vi "Flow Module (Main).vi"(7 "Name of Parent Panel":string="Main.vi", 9 "New Center Coords":T1={"Horizontal"=470, "Vertical"=200}, 10 "Config":variant, 11 "Main UI Message Queue":refnum<queue>) -> ()   [LabVIEW 2018, in "Flow Module.lvlib"]
doc: "This Continuous Measurement sample project is based on the Queued Message Handler template.\n\nThe Event Handling Loop generates messages based on user interface actions.\n\nThe Message Handling Loop processes messages generated by the Event Handling Loop, or by other messages. There are also Acquisition and Logging message handling loop subVIs, and a chart updating loop."
uses:
  Flow Module.lvlib
  support/Message Queue/Message Cluster.ctl
  <vilib>/Utility/miscctls.llb/LVPoint32TypeDef.ctl
  controls/UI State.ctl
  Feed Module/Controls/Flow Module Config Cluster.ctl
  Feed Module/Controls/Flow Module Settings Cluster.ctl
  Mettler Toledo/Controls/Settings Cluster.ctl
  Feed Module/Controls/Flow Module State Cluster.ctl
  Feed Module/Controls/Flow Module Display.ctl
  support/Message Queue/Enqueue Message (Single).vi
  support/User Event - Stop/User Event - Stop.lvlib
  support/Message Queue/Message Queue.lvlib
  support/Support Library.lvlib
  Measure Instrument/Flow Module Engine.lvlib
  Mettler Toledo/Mettler Toledo.lvlib
  support/Command Log VIs/Command Logging.lvlib
panel:
  in  "Settings Button":bool
  out "C":dbl format="%5.2f"
  out "kg/m^3":dbl format="%6.1f"
  out "ScanCode":i16
  out "g/min":dbl format="%4.2f"
  out "Log File path":path
  out "Status":string
  in  "Exit":bool
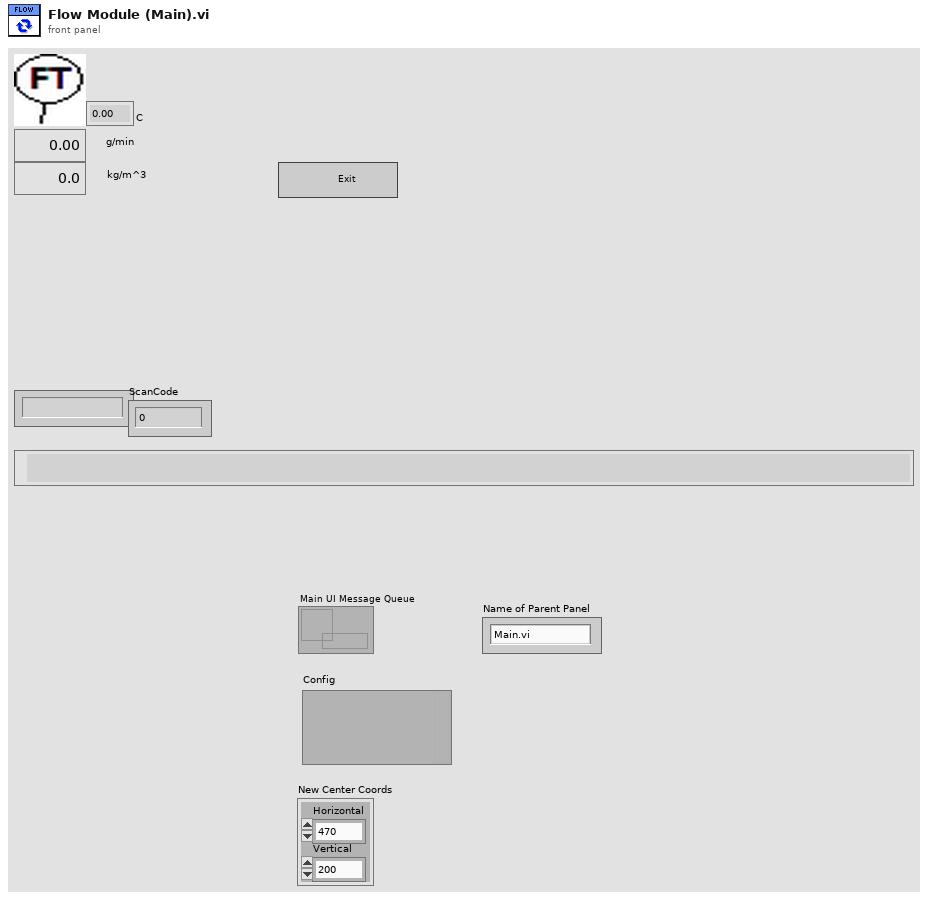
[diagram p1: front panel]
types:
  T1 = typedef "LVPoint32TypeDef.ctl" = cluster{"Horizontal":i32, "Vertical":i32}
  T2 = typedef "Flow Module.lvlib/Flow Module State Cluster.ctl" = cluster{"Flow Module Config":T3}
  T3 = typedef "Flow Module.lvlib/Flow Module Config Cluster.ctl" = cluster{"GUID":string, "Drop Coords":T1, "Process Name":string, "Queue Name":string, "Settings":T4, "Load Count":i32}
  T4 = typedef "Flow Module.lvlib/Flow Module Settings Cluster.ctl" = cluster{"Cycle Period":dbl, "Bronkhorst M13":T5, "Flow Meter Type":string, "Bronkhorst M14":T5}
  T5 = typedef "Mettler Toledo.lvlib/Settings Cluster.ctl" = cluster{"VISA resource name":refnum<visa-resource-name>, "Simulated?":bool}
  T6 = typedef "UI State.ctl" = enum16{"Idle", "Acquiring and Logging", "Waiting for Exit", "Waiting for Exit (Acq Stopped)", "Waiting for Exit (Log Stopped)", "Waiting for Stop", "Waiting for Stop (Acq Stopped)", "Waiting for Stop (Log Stopped)"}
  T7 = typedef "Flow Module.lvlib/Flow Message Queues.ctl" = cluster{"Flow UI":refnum<queue>, "Flow Engine":refnum<queue>, "Flow Display":refnum<queue>}
  T8 = typedef "Flow Module.lvlib/Flow Module Display.ctl" = cluster{"Flow Value":dbl, "Cycle Period":dbl, "Density":dbl, "Temp":dbl}
  T9 = cluster{"Shift":bool, "Ctrl":bool, "Alt":bool, "Cmd":bool, "Opt":bool}
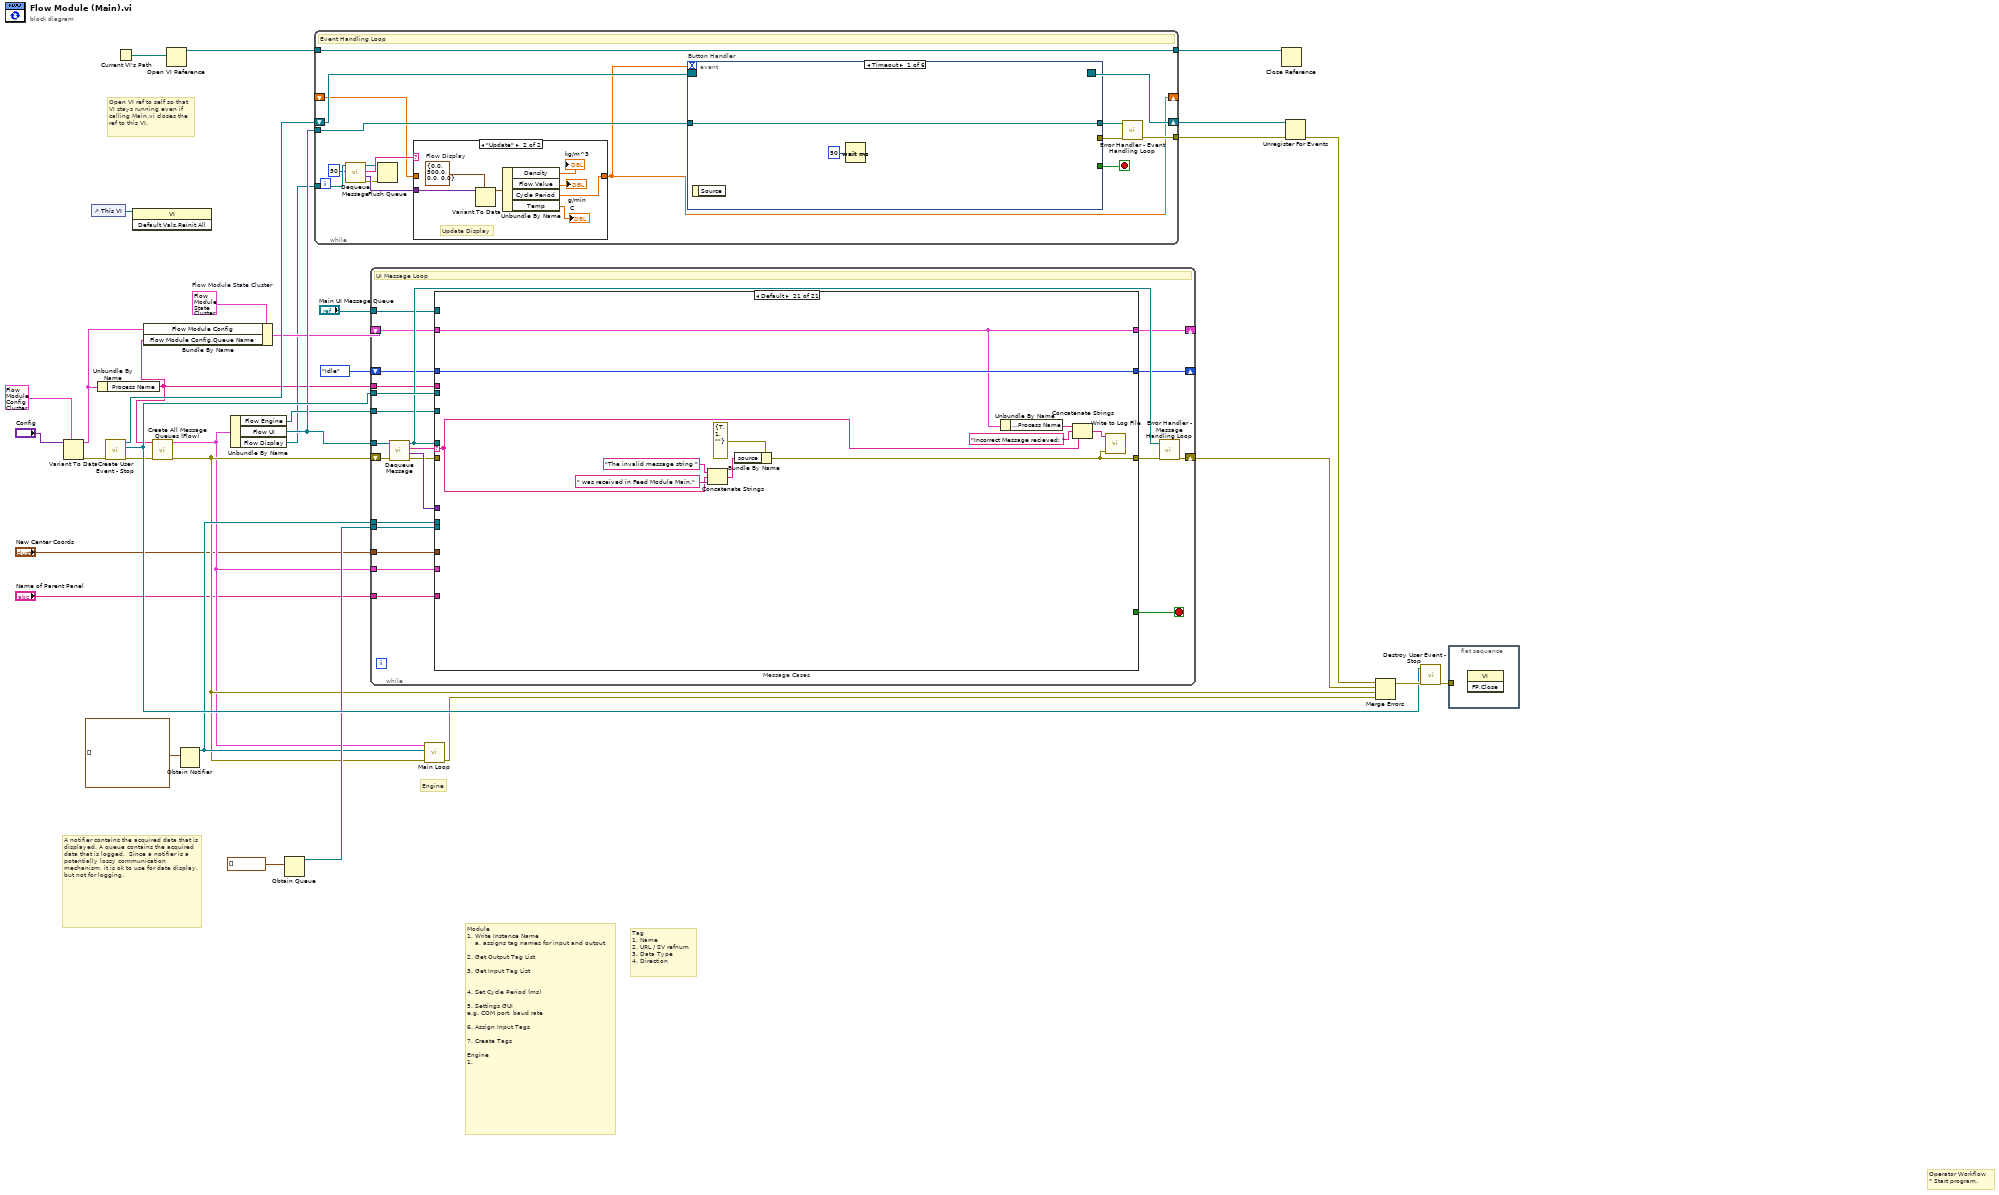
[diagram p0: block diagram]
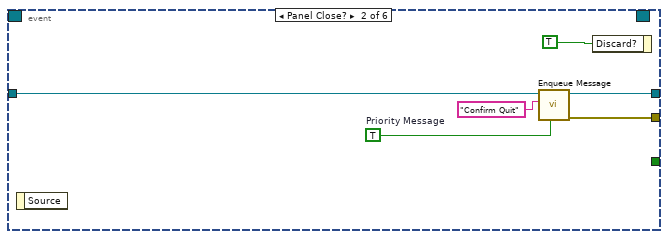
[diagram p3: hidden frame]
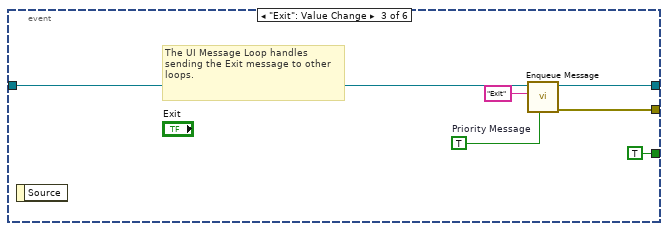
[diagram p4: hidden frame]
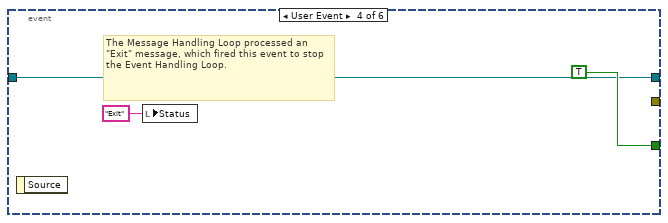
[diagram p5: hidden frame]
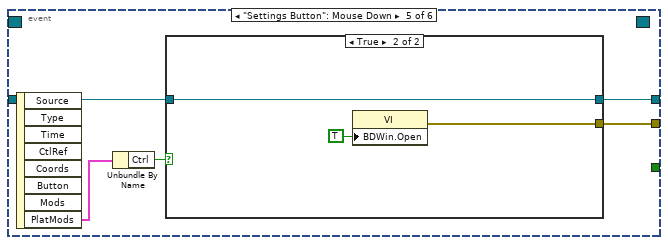
[diagram p6: hidden frame]
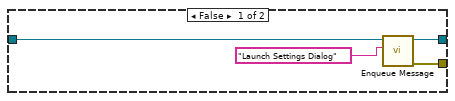
[diagram p7: hidden frame]
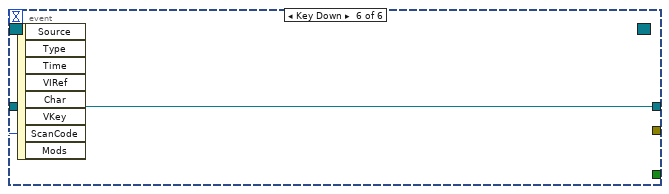
[diagram p8: hidden frame]
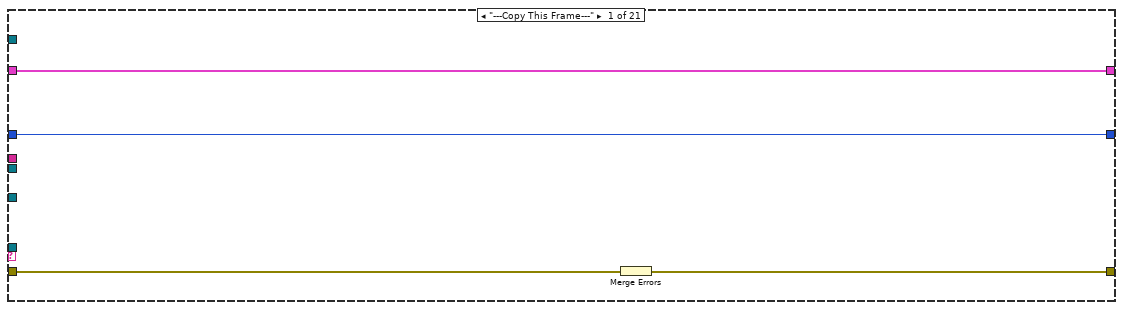
[diagram p9: hidden frame]
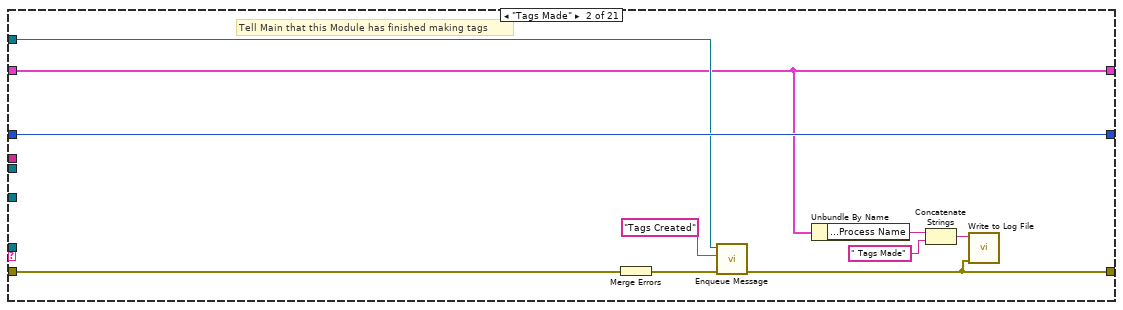
[diagram p10: hidden frame]
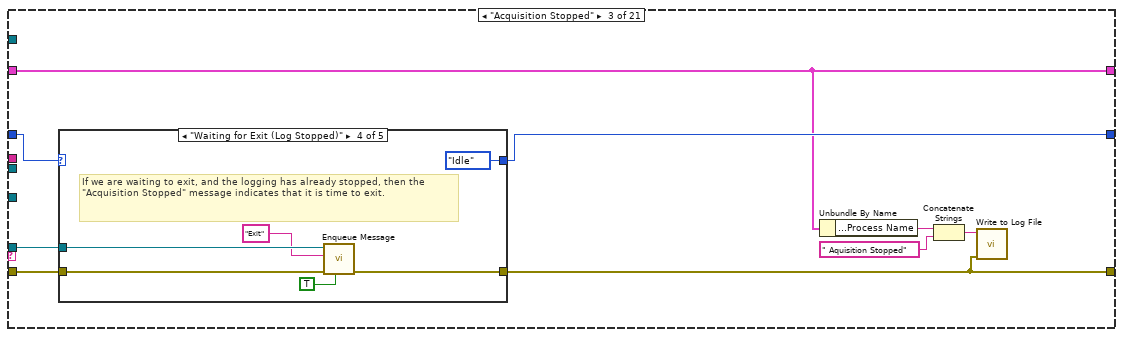
[diagram p11: hidden frame]
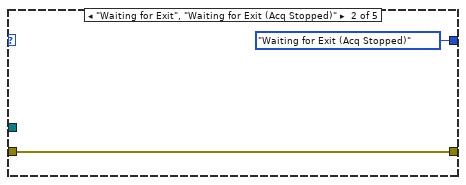
[diagram p13: hidden frame]
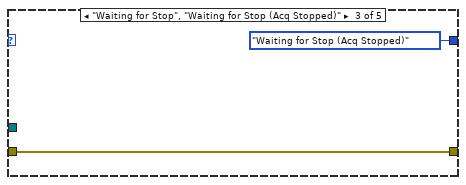
[diagram p14: hidden frame]
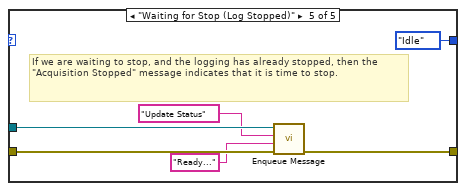
[diagram p15: hidden frame]
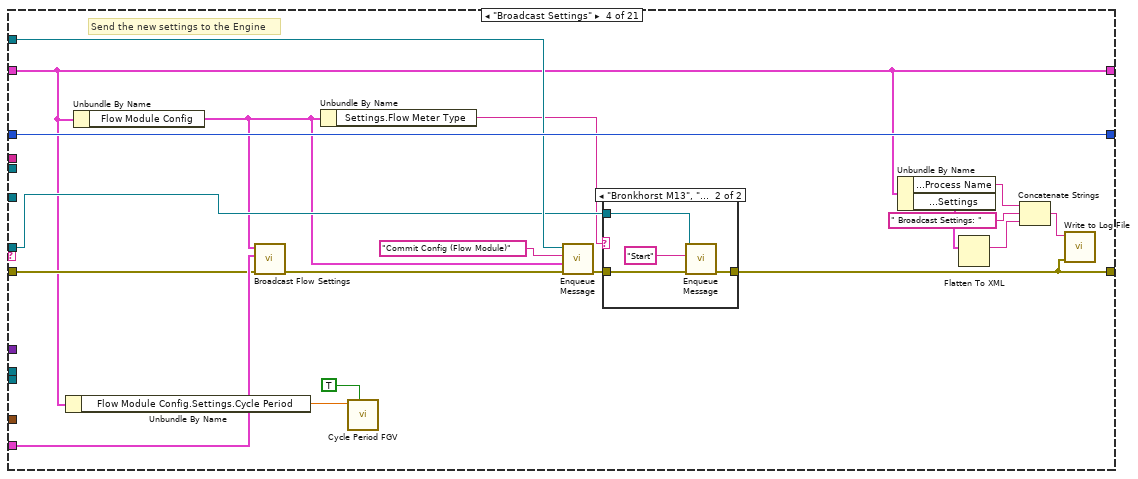
[diagram p16: hidden frame]
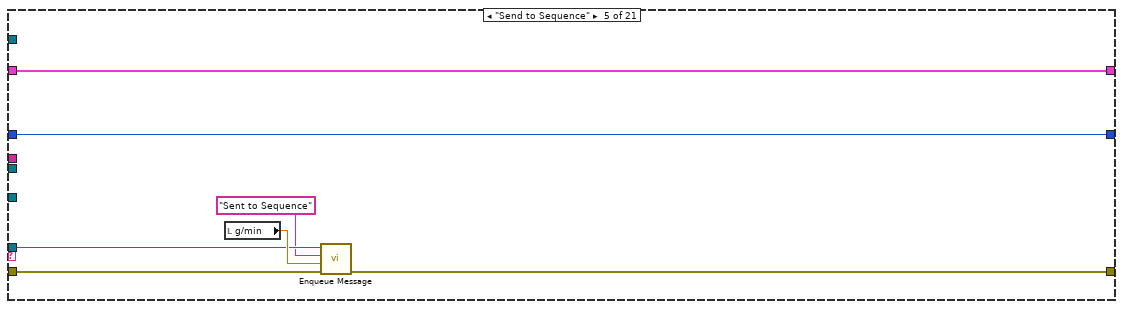
[diagram p18: hidden frame]
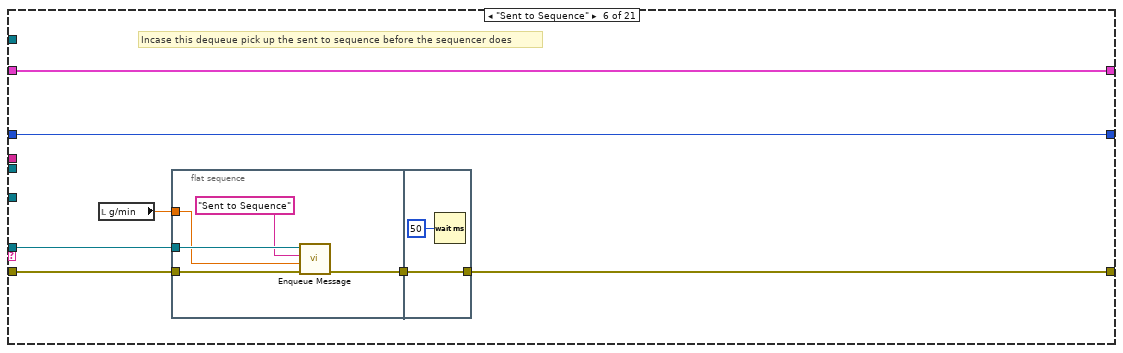
[diagram p19: hidden frame]
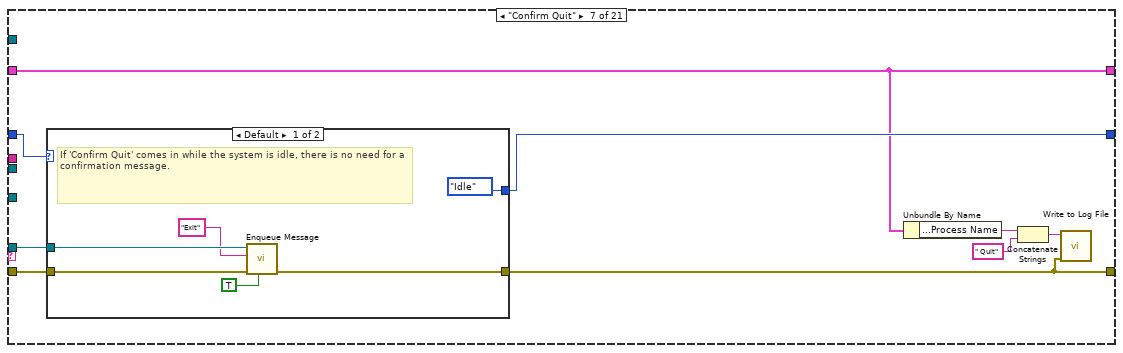
[diagram p20: hidden frame]
diagram:
  w2 = T2 {"Flow Module Config"={"GUID"="PID1-Mettler Toledo Scale 1", "Drop Coords"={"Horizontal"=0, "Vertical"=0}, "Process Name"="PID1-Setpoint", "Queue Name"="", "Settings"={"Cycle Period"=500.0, "Bronkhorst M13"={"VISA resource name"="", "Simulated?"=FALSE}, "Flow Meter Type"="", "Bronkhorst M14"={"VISA resource name"="", "Simulated?"=FALSE}}, "Load Count"=0}}  # Flow Module State Cluster
  # "Open VI ref to self so that\nVI stays running even if\ncalling Main.vi closes the\nref to this VI."
  # "Engine"
  # "Operator Workflow\n* Start program."
  # "Module \n1. Write Instance Name\n    a. assigns tag names for input and output\n\n2. Get Output Tag List\n\n3. Get Input Tag List\n\n\n4. Set Cycle Period (ms)\n\n5. Settings GUI\ne.g. COM port, baud rate\n\n6. Assign Input Tags\n\n7. Create Tags\n\nEngine\n1."
  # "Tag\n1. Name\n2. URL / SV refnum\n3. Data Type\n4. Direction"
  # "A notifier contains the acquired data that is displayed. A queue contains the acquired data that is logged.  Since a notifier is a potentially lossy communication mechanism, it is ok to use for data display, but not for logging."
  n1 = Variant To Data(type=T3 {"GUID"="", "Drop Coords"={"Horizontal"=0, "Vertical"=0}, "Process Name"="", "Queue Name"="", "Settings"={"Cycle Period"=500.0, "Bronkhorst M13"={"VISA resource name"="", "Simulated?"=FALSE}, "Flow Meter Type"="", "Bronkhorst M14"={"VISA resource name"="", "Simulated?"=FALSE}}, "Load Count"=0} ("Feed Module Config"), Variant="Config") -> (data=w11:T3, error out=w15:errorcluster)  [unwired: 1 in]
  n2 = control-ref of="This VI"() -> (w10:refnum<vi>)
  n3 = Unbundle By Name(w11) -> ("Process Name"=w1:string)
  n4 = call "Create User Event - Stop.vi"("error in (no error)"=w15) -> ("error out"=w8:errorcluster, "User Event - Stop"=w30:refnum<user-event>, "Stop Event Registration Refnum"=w31:refnum<event-registration>)  [unwired: 8 in]
  n5 = Current VI's Path() -> (path=w17:path)
  n6 = invoke class="VI" method="Default Vals.Reinit All"(reference=w10) -> ()  [unwired: 2 in, 3 out]
  n7 = Bundle By Name(cluster=w2, "Flow Module Config"=w11, "Flow Module Config.Queue Name"=w1) -> (w16:T2)
  n8 = call "Create All Message Queues (Flow).vi"("error in (no error)"=w8, "Process Name"=w1) -> ("error out"=w7:errorcluster, "Message Queues"=w6:T7)  [unwired: 8 in]
  n9 = Open VI Reference(vi path=w17) -> (vi reference=w18:refnum<vi>)  [unwired: 5 in, 1 out]
  n10 = Obtain Notifier(notification data type=waveform(dbl)[] []) -> (notifier out=w20:refnum<notifier>)  [unwired: 3 in, 2 out]
  n11 = Unbundle By Name(w6) -> ("Flow Engine"=w23:refnum<queue>, "Flow UI"=w27:refnum<queue>, "Flow Display"=w12:refnum<queue>)
  n12 = Obtain Queue(element data type=waveform(dbl)[] []) -> (queue out=w22:refnum<queue>)  [unwired: 4 in, 2 out]
  n13 = while {
    tunnel: w27 -> [w44]
    tunnel: [w46] -> w33
    shift-right: [w45] -> w28
    shift-left: w31 -> [w50]
    tunnel: [w43] -> w19
    tunnel: w18 -> [w43]
    tunnel: w12 -> [w42]
    shift-right: [w39] -> _
    shift-left: _ -> [w38]
    stop <- w49 stop-if-true
    # "Event Handling Loop"
    n14 = call "Dequeue Message.vi"("timeout in ms (-1)"=50, "Message Queue"=w42) -> ("error out"=w35:errorcluster, "Message Data"=w40:variant, "Message"=w41:string, "dup Message Queue"=w36:refnum<queue>)  [unwired: 6 in]
    n15 = Flush Queue(queue=w36, error in (no error)=w35) -> ()  [unwired: 3 out]
    n16 = case shown="\"Update\"" w41 {
      tunnel: w40 -> [_ w58]
      tunnel: [w51 w55] -> w39
      tunnel: w38 -> [w51 _]
      frame "False", Default {
      }
      frame "Update" {
        w54 = T8 {"Flow Value"=0.0, "Cycle Period"=500.0, "Density"=0.0, "Temp"=0.0}  # Flow Display
        # "Update Display"
        n17 = Variant To Data(type=w54, Variant=w58) -> (data=w57:T8)  [unwired: 1 in, 1 out]
        n18 = Unbundle By Name(w57) -> ("Density"=→"kg/m^3":dbl, "Flow Value"=→"g/min":dbl, "Cycle Period"=w55:dbl, "Temp"=→"C":dbl)
      }
    }
    n19 = event "Button Handler" shown="[0] Timeout" {
      selector: w50 -> [_ _ _ _ _ _]
      dyn-events: [_ _ _ _ _ _] -> w45
      timeout: w39 -> [_ _ _ _ _ _]
      tunnel: [_ _ TRUE ("Discard?") TRUE ("Discard?") _ _] -> w49
      tunnel: w44 -> [w60 w63 w67 w73 w78 w88]
      tunnel: [_ w61 w72 _ w80 _] -> w47
      tunnel: [w60 w62 w70 w73 w79 w88] -> w48
      event Timeout {
        n20 = event-data() -> ()  [unwired: 1 in, 1 out]
        n21 = Wait (ms)(milliseconds to wait=u32 50) -> ()  [unwired: 1 out]
      }
      event Panel Close? {
        w64 = TRUE  # Priority Message
        n22 = event-data() -> ()  [unwired: 1 in, 1 out]
        n23 = call-poly "Enqueue Message.vi"("Priority Message? (F)"=w64, "Message"="Confirm Quit", "Message Queue"=w63) -> ("error out"=w61:errorcluster, "dup Message Queue"=w62:refnum<queue>)  [unwired: 7 in]
        n24 = event-data("Discard?"=TRUE) -> ()  [unwired: 1 in, 1 out]
      }
      event "Exit": Value Change {
        w68 = TRUE  # Priority Message
        # "The UI Message Loop handles sending the Exit message to other loops."
        n25 = event-data() -> ()  [unwired: 1 in, 1 out]
        n26 = call-poly "Enqueue Message.vi"("Priority Message? (F)"=w68, "Message"="Exit", "Message Queue"=w67) -> ("error out"=w72:errorcluster, "dup Message Queue"=w70:refnum<queue>)  [unwired: 7 in]
      }
      event User Event {
        # "The Message Handling Loop processed an \"Exit\" message, which fired this event to stop the Event Handling Loop."
        n27 = event-data() -> ()  [unwired: 1 in, 1 out]
        n28 = local write "Status"("Exit" ("Exit String")) -> ()
      }
      event "Settings Button": Mouse Down {
        n29 = event-data() -> ("PlatMods"=w77:T9)  [unwired: 1 in, 7 out]
        n30 = Unbundle By Name(w77) -> ("Ctrl"=w76:bool)
        n31 = case shown="True" w76 {
          tunnel: [w84 w85] -> w80
          tunnel: [w83 w86] -> w79
          tunnel: w78 -> [w82 w86]
          frame False {
            n32 = call-poly "Enqueue Message.vi"("Message"="Launch Settings Dialog", "Message Queue"=w82) -> ("error out"=w84:errorcluster, "dup Message Queue"=w83:refnum<queue>)  [unwired: 8 in]
          }
          frame True {
            n33 = property class="VI"("BDWin.Open"=TRUE ("Block Diagram Window:Open")) -> (error out=w85:errorcluster)  [unwired: 2 in, 1 out]
          }
        }
      }
      event Key Down {
        n34 = event-data() -> ("ScanCode"=→"ScanCode":i16)  [unwired: 1 in, 7 out]
      }
    }
    n35 = call "Error Handler - Event Handling Loop.vi"("error in (no error)"=w47, "Message Queue"=w48) -> ("dup error in"=w46:errorcluster)  [unwired: 8 in, 1 out]
  }
  n36 = while {
    tunnel: w27 -> [w106]
    tunnel: w30 -> [w110]
    shift-right: [w102] -> w34
    shift-left: w7 -> [w109]
    shift-right: [w93] -> _
    shift-left: w16 -> [w95]
    tunnel: w20 -> [w105]
    tunnel: w22 -> [w104]
    shift-right: [w99] -> _
    shift-left: UI_State."Idle" ("UI State") -> [w100]
    tunnel: w23 -> [w98]
    tunnel: w6 -> [w97]
    tunnel: "Main UI Message Queue" -> [w94]
    tunnel: w1 -> [w92]
    tunnel: "New Center Coords" -> [w91]
    tunnel: "Name of Parent Panel" -> [w90]
    stop <- w111 stop-if-true
    # "UI Message Loop"
    n37 = call "Dequeue Message.vi"("error in (no error)"=w109, "Message Queue"=w106) -> ("error out"=w96:errorcluster, "Message Data"=w107:variant, "Message"=w108:string, "dup Message Queue"=w101:refnum<queue>)  [unwired: 6 in]
    n38 = case "Message Cases" shown="Default" w108 {
      selector: w108 -> [_ _ _ _ _ _ _ _ _ _ _ _ _ _ _ _ _ _ _ _ w436]
      tunnel: w101 -> [_ _ w131 w163 w178 w186 w205 _ w246 w260 w282 _ w321 w338 w355 w383 _ _ w425 _ _]
      tunnel: w96 -> [w115 w125 w132 w167 w181 w188 w204 w230 w241 w264 w281 w307 w317 w335 w356 w382 w389 w408 w420 w434 _]
      tunnel: [w114 w117 w127 w156 w180 w187 w199 w231 w236 w251 w266 w307 w309 w328 w351 w378 w394 w401 w412 w435 w437] -> w103
      tunnel: [_ _ _ _ _ _ _ _ _ _ TRUE _ _ _ _ _ _ _ _ _ _] -> w111
      tunnel: w107 -> [_ _ _ _ _ _ _ w233 _ w263 w271 _ _ _ _ _ _ _ _ w433 _]
      tunnel: w110 -> [_ _ _ _ _ _ _ _ _ _ w292 _ _ _ _ _ _ _ _ _ _]
      tunnel: w95 -> [w112 w116 w126 w155 w182 w189 w198 w228 w235 w250 w265 w304 w308 w340 w350 w377 w387 w400 w411 w428 w442]
      tunnel: w105 -> [_ _ _ _ _ _ _ _ _ _ w290 _ _ _ _ _ _ _ _ _ _]
      tunnel: w104 -> [_ _ _ _ _ _ _ _ _ _ w286 _ _ _ _ _ _ _ _ _ _]
      tunnel: w100 -> [w113 w124 w134 w171 w183 w190 w206 w229 w242 w255 w279 _ _ w344 w358 _ _ _ w421 w429 w446]
      tunnel: [w113 w124 w133 w171 w183 w190 w203 w229 w243 w255 w278 UI_State."Idle" ("UI State") UI_State."Idle" ("UI State") w344 w357 UI_State."Acquiring and Logging" ("UI State") UI_State."Acquiring and Logging" ("UI State") UI_State."Acquiring and Logging" ("UI State") w422 w429 w446] -> w99
      tunnel: w98 -> [_ _ _ _ _ _ _ _ _ _ w285 _ _ _ _ _ w392 w406 w419 _ _]
      tunnel: w97 -> [_ _ _ w170 _ _ _ _ _ _ _ _ _ _ _ _ _ _ _ _ _]
      tunnel: w94 -> [_ w121 _ w164 _ _ _ _ _ _ w270 _ _ w341 _ _ _ _ _ _ _]
      tunnel: [w112 w116 w126 w155 w182 w189 w198 w228 w235 w250 w265 w304 w308 w329 w350 w377 w387 w400 w411 w428 w442] -> w93
      tunnel: w92 -> [_ _ _ _ _ _ _ _ _ _ _ _ w315 _ _ _ _ w405 _ _ _]
      tunnel: w91 -> [_ _ _ _ _ _ _ _ _ _ _ _ w314 _ _ _ _ _ _ _ _]
      tunnel: w90 -> [_ _ _ _ _ _ _ _ _ _ _ _ w313 _ _ _ _ _ _ _ _]
      frame "---Copy This Frame---" {
        # "Duplicate this frame when creating new messages.  Change this comment in the duplicated frame to describe this message."
        n39 = Merge Errors(w115) -> (w114:errorcluster)
      }
      frame "Tags Made" {
        # "Tell Main that this Module has finished making tags"
        # "Duplicate this frame when creating new messages.  Change this comment in the duplicated frame to describe this message."
        n40 = Merge Errors(w125) -> (w122:errorcluster)
        n41 = call-poly "Enqueue Message.vi"("error in (no error)"=w122, "Message"="Tags Created", "Message Queue"=w121) -> ("error out"=w117:errorcluster)  [unwired: 7 in, 1 out]
        n42 = Unbundle By Name(w116) -> ("Flow Module Config.Process Name"=w120:string)
        n43 = Concatenate Strings(w120, " Tags Made" ("text")) -> (w118:string)
        n44 = call "Write to Log File.vi"("error in"=w117, "text"=w118) -> ()  [unwired: 9 in, 1 out]
      }
      frame "Acquisition Stopped" {
        # "Logic for determining what action to take when the acquisition has stopped."
        n45 = case shown="\"Waiting for Exit (Log Stopped)\"" w134 {
          selector: w134 -> [w136 _ _ _ _]
          tunnel: [w136 UI_State."Waiting for Exit (Acq Stopped)" ("UI State") UI_State."Waiting for Stop (Acq Stopped)" ("UI State") UI_State."Idle" ("UI State") UI_State."Idle" ("UI State")] -> w133
          tunnel: w132 -> [w135 w137 w139 w145 w151]
          tunnel: [w135 w137 w139 w144 w150] -> w127
          tunnel: w131 -> [_ _ _ w143 w149]
          frame Default {
          }
          frame "Waiting for Exit", "Waiting for Exit (Acq Stopped)" {
          }
          frame "Waiting for Stop", "Waiting for Stop (Acq Stopped)" {
          }
          frame "Waiting for Exit (Log Stopped)" {
            # "If we are waiting to exit, and the logging has already stopped, then the \"Acquisition Stopped\" message indicates that it is time to exit."
            n46 = call-poly "Enqueue Message.vi"("Priority Message? (F)"=TRUE, "error in (no error)"=w145, "Message"="Exit", "Message Queue"=w143) -> ("error out"=w144:errorcluster)  [unwired: 6 in, 1 out]
          }
          frame "Waiting for Stop (Log Stopped)" {
            # "If we are waiting to stop, and the logging has already stopped, then the \"Acquisition Stopped\" message indicates that it is time to stop."
            n47 = call-poly "Enqueue Message.vi"("error in (no error)"=w151, "Message Data"="Ready..." ("Message"), "Message"="Update Status", "Message Queue"=w149) -> ("error out"=w150:errorcluster)  [unwired: 6 in, 1 out]
          }
        }
        n48 = Unbundle By Name(w126) -> ("Flow Module Config.Process Name"=w130:string)
        n49 = Concatenate Strings(w130, " Aquisition Stopped" ("text")) -> (w128:string)
        n50 = call "Write to Log File.vi"("error in"=w127, "text"=w128) -> ()  [unwired: 9 in, 1 out]
      }
      frame "Broadcast Settings" {
        # "Send the new settings to the Engine"
        # "Send the 'Update Settings' message to the Logging and Acquisition message loops."
        n51 = Unbundle By Name(w155) -> ("Flow Module Config.Settings.Cycle Period"=w168:dbl)
        n52 = Unbundle By Name(w155) -> ("Flow Module Config"=w160:T3)
        n53 = call "Broadcast Flow Settings.vi"("error in (no error)"=w167, "Message Queues"=w170, "Flow Module Config"=w160) -> ("error out"=w165:errorcluster)  [unwired: 8 in]
        n54 = Unbundle By Name(w160) -> ("Settings.Flow Meter Type"=w161:string)
        n55 = call "Cycle Period FGV.vi"("Write"=TRUE, "Cycle Period In (ms)"=w168) -> ()  [unwired: 8 in, 2 out]
        n56 = call-poly "Enqueue Message.vi"("error in (no error)"=w165, "Message Data"=w160, "Message"="Commit Config (Flow Module)", "Message Queue"=w164) -> ("error out"=w162:errorcluster)  [unwired: 6 in, 1 out]
        n57 = case shown="\"Bronkhorst M13\", \"Bronkhorst M14\"" w161 {
          tunnel: w163 -> [_ w175]
          tunnel: w162 -> [w172 w174]
          tunnel: [w172 w173] -> w156
          frame "False", Default {
          }
          frame "Bronkhorst M13", "Bronkhorst M14" {
            n58 = call-poly "Enqueue Message.vi"("error in (no error)"=w174, "Message"="Start", "Message Queue"=w175) -> ("error out"=w173:errorcluster)  [unwired: 7 in, 1 out]
          }
        }
        n59 = Unbundle By Name(w155) -> ("Flow Module Config.Process Name"=w159:string, "Flow Module Config.Settings"=w154:T4)
        n60 = Flatten To XML(anything=w154) -> (xml string=w153:string)
        n61 = Concatenate Strings(w159, " Broadcast Settings: " ("text"), w153) -> (w157:string)
        n62 = call "Write to Log File.vi"("error in"=w156, "text"=w157) -> ()  [unwired: 9 in, 1 out]
      }
      frame "Send to Sequence" {
        n63 = local read "g/min"() -> (w179:dbl)
        n64 = call-poly "Enqueue Message.vi"("error in (no error)"=w181, "Message Data"=w179, "Message"="Sent to Sequence", "Message Queue"=w178) -> ("error out"=w180:errorcluster)  [unwired: 6 in, 1 out]
      }
      frame "Sent to Sequence" {
        # "Incase this dequeue pick up the sent to sequence before the sequencer does"
        n65 = local read "g/min"() -> (w184:dbl)
        n66 = flat-sequence {
          tunnel: w188 -> [w195]
          tunnel: w186 -> [w193]
          tunnel: [w194] -> w185
          tunnel: w184 -> [w191]
          tunnel: [w197] -> w187
          tunnel: w185 -> [w197]
          frame #0 {
            n67 = call-poly "Enqueue Message.vi"("error in (no error)"=w195, "Message Data"=w191, "Message"="Sent to Sequence", "Message Queue"=w193) -> ("error out"=w194:errorcluster)  [unwired: 6 in, 1 out]
          }
          frame #1 {
            n68 = Wait (ms)(milliseconds to wait=u32 50) -> ()  [unwired: 1 out]
          }
        }
      }
      frame "Confirm Quit" {
        # "Confirm Quit - Message that can confirm whether or not the user wants to exit the application."
        n69 = case shown="Default" w206 {
          tunnel: w205 -> [w211 w217]
          tunnel: w204 -> [w210 w215]
          tunnel: [w207 w214] -> w199
          tunnel: [UI_State."Idle" ("UI State") w213] -> w203
          frame Default {
            # "If 'Confirm Quit' comes in while the system is idle, there is no need for a confirmation message."
            n70 = call-poly "Enqueue Message.vi"("Priority Message? (F)"=TRUE, "error in (no error)"=w210, "Message"="Exit", "Message Queue"=w211) -> ("error out"=w207:errorcluster)  [unwired: 6 in, 1 out]
          }
          frame "Acquiring and Logging" {
            n71 = Two Button Dialog(message="Are you sure you want to quit while the acquisition is running?" ("Confirm Quit Message"), 1:"No" ("No"), 2:"Yes" ("Yes")) -> (T button?=w216:bool)
            n72 = case shown="True" w216 {
              tunnel: w217 -> [_ w227]
              tunnel: w215 -> [w221 w226]
              tunnel: [w221 w225] -> w214
              tunnel: [UI_State."Acquiring and Logging" ("UI State") UI_State."Waiting for Exit" ("UI State")] -> w213
              frame False {
                # "User did not want to quit."
              }
              frame True {
                n73 = call-poly "Enqueue Message.vi"("error in (no error)"=w226, "Message"="Exit", "Message Queue"=w227) -> ("error out"=w225:errorcluster)  [unwired: 7 in, 1 out]
              }
            }
          }
        }
        n74 = Unbundle By Name(w198) -> ("Flow Module Config.Process Name"=w202:string)
        n75 = Concatenate Strings(w202, " Quit" ("text")) -> (w200:string)
        n76 = call "Write to Log File.vi"("error in"=w199, "text"=w200) -> ()  [unwired: 9 in, 1 out]
      }
      frame "Display Log File Path" {
        n77 = Variant To Data(error in=w230, type=path "", Variant=w233) -> (data=→"Log File path":path, error out=w231:errorcluster)
      }
      frame "E-Stop" {
        # "Doesn't really do anything because this is just a read module"
        # "Message Acquisition and Logging loops to stop"
        # "Stop the pumps."
        n78 = call-poly "Enqueue Message.vi"("error in (no error)"=w241, "Message Data"="Ready..." ("Ready..."), "Message"="Update Status", "Message Queue"=w246) -> ("error out"=w240:errorcluster)  [unwired: 6 in, 1 out]
        n79 = case shown="\"Waiting for Exit\"" w242 {
          selector: w242 -> [_ w248]
          tunnel: [UI_State."Waiting for Stop" ("UI State") w248] -> w243
          frame Default {
          }
          frame "Waiting for Exit" {
          }
        }
        n80 = Merge Errors(w240) -> (w236:errorcluster)
        n81 = Unbundle By Name(w235) -> ("Flow Module Config.Process Name"=w239:string)
        n82 = Concatenate Strings(w239, " E-STOP" ("text")) -> (w237:string)
        n83 = call "Write to Log File.vi"("error in"=w236, "text"=w237) -> ()  [unwired: 9 in, 1 out]
      }
      frame "Error" {
        # "Exit on error"
        # "Error - Check the error message data and respond accordingly. This message is sent by the \"Error Handler\" VIs at the end of each loop in this application."
        n84 = Variant To Data(error in=w264, type=errorcluster {"status"=FALSE, "code"=0, "source"=""} ("error out"), Variant=w263) -> (data=w261:errorcluster, error out=w257:errorcluster)
        n85 = call <vilib>:"General Error Handler.vi"("error in (no error)"=w261) -> ("message"=w249:string)  [unwired: 10 in, 4 out]
        n86 = call-poly "Enqueue Message.vi"("Priority Message? (F)"=TRUE, "Message"="Exit", "Message Queue"=w260) -> ("error out"=w256:errorcluster)  [unwired: 7 in, 1 out]
        n87 = Merge Errors(w256, w257) -> (w251:errorcluster)
        n88 = Unbundle By Name(w250) -> ("Flow Module Config.Process Name"=w254:string)
        n89 = Concatenate Strings(w254, " Error: " ("text"), w249) -> (w252:string)
        n90 = call "Write to Log File.vi"("error in"=w251, "text"=w252) -> ()  [unwired: 9 in, 1 out]
      }
      frame "Exit" {
        w274 = TRUE  # Delete Module?
        # "Don't check the error outs. The acquisition and logging queues may have already been released."
        # "Close references owned by the Main VI."
        # "Stop the VI"
        # "Exit - Fire the User Event to stop the Event Handling Loop.  Also send Exit messages to the Acquisition and Logging loops."
        n91 = Build Array(w285) -> (w284:refnum<queue>[])
        n92 = Variant To Data(type=w274, Variant=w271) -> (data=w273:bool, error out=w275:errorcluster)  [unwired: 1 in]
        n93 = Select(t=w274, s=w275, f=w273) -> (s? t:f=w272:bool)
        n94 = for {
          tunnel: w284 -> [w301] mode=indexing
          # "Stop Logging and Exit"
          n95 = call-poly "Enqueue Message.vi"("Message"="Stop", "Message Queue"=w301) -> ("dup Message Queue"=w302:refnum<queue>)  [unwired: 8 in, 1 out]
          n96 = call-poly "Enqueue Message.vi"("Message"="Exit", "Message Queue"=w302) -> ()  [unwired: 8 in, 2 out]
        }
        n97 = case "Don't enqueue Delete Module if opening campaign because it\nwill already have been deleted and new config loaded and we create\na race condition." shown="True" w272 {
          tunnel: w270 -> [_ w296]
          tunnel: w265 -> [_ w295]
          frame False {
          }
          frame True {
            n98 = Unbundle By Name(w295) -> ("Flow Module Config.GUID"=w294:string)
            n99 = call-poly "Enqueue Message.vi"("Message Data"=w294, "Message"="Delete Module", "Message Queue"=w296) -> ()  [unwired: 7 in, 2 out]
          }
        }
        n100 = call-poly "Enqueue Message.vi"("error in (no error)"=w281, "Message Data"="Ready..." ("Ready..."), "Message"="Update Status", "Message Queue"=w282) -> ("error out"=w280:errorcluster, "dup Message Queue"=w277:refnum<queue>)  [unwired: 6 in]
        n101 = Release Queue(queue=w277, error in (no error)=w280) -> (error out=w289:errorcluster)  [unwired: 1 in, 2 out]
        n102 = Release Notifier(notifier=w290, error in (no error)=w289) -> (error out=w288:errorcluster)  [unwired: 1 in, 2 out]
        n103 = call "Fire User Event - Stop.vi"("User Event - Stop"=w292) -> ("error out"=w291:errorcluster)  [unwired: 10 in]
        n104 = Release Queue(queue=w286, error in (no error)=w288) -> (error out=w287:errorcluster)  [unwired: 1 in, 2 out]
        n105 = case shown="Default" w279 {
          selector: w279 -> [_ w299]
          tunnel: [UI_State."Waiting for Stop" ("UI State") w299] -> w278
          frame Default {
          }
          frame "Waiting for Exit" {
          }
        }
        n106 = Merge Errors(w291, w287) -> (w266:errorcluster)
        n107 = Unbundle By Name(w265) -> ("Flow Module Config.Process Name"=w269:string)
        n108 = Concatenate Strings(w269, " Exit" ("text")) -> (w267:string)
        n109 = call "Write to Log File.vi"("error in"=w266, "text"=w267) -> ()  [unwired: 9 in, 1 out]
      }
      frame "Init UI Refs" {
        # "Init UI Refs - Store control references for UI controls.  Also enable/disable controls appropriately."
        n110 = property class="VI"("Front Panel.Closeable"=TRUE ("Front Panel Window:Closeable")) -> ()  [unwired: 2 in, 2 out]
      }
      frame "Initialize" {
        # "Initialize - Get configuration settings, then message the UI to initialize, and broadcast the settings to the other message loops."
        n111 = property class="VI" props=["FP.State"]() -> (reference out=w316:refnum<vi>)  [unwired: 2 in, 2 out]
        n112 = call-poly "Enqueue Message.vi"("error in (no error)"=w317, "Message"="Init UI Refs", "Message Queue"=w321) -> ("error out"=w319:errorcluster, "dup Message Queue"=w320:refnum<queue>)  [unwired: 7 in]
        n113 = call "Make Child and Move.vi"("Process Name"=w315, "Name of Parent Panel"=w313, "New Center Coords"=w314, "VI in"=w316) -> ()  [unwired: 8 in]
        n114 = call-poly "Enqueue Message.vi"("error in (no error)"=w319, "Message"="Broadcast Settings", "Message Queue"=w320) -> ("error out"=w327:errorcluster, "dup Message Queue"=w326:refnum<queue>)  [unwired: 7 in]
        n115 = call-poly "Enqueue Message.vi"("error in (no error)"=w327, "Message Data"="Ready..." ("Ready..."), "Message"="Update Status", "Message Queue"=w326) -> ("error out"=w309:errorcluster)  [unwired: 6 in, 1 out]
        n116 = Unbundle By Name(w308) -> ("Flow Module Config.Process Name"=w312:string)
        n117 = Concatenate Strings(w312, " Initialize" ("text")) -> (w310:string)
        n118 = call "Write to Log File.vi"("error in"=w309, "text"=w310) -> ()  [unwired: 9 in, 1 out]
      }
      frame "Launch Settings Dialog" {
        # "Keep track of the # of times the dialog has been opened"
        # "Launch the Settings Dialog when the user clicks the 'Settings' button."
        n119 = Unbundle By Name(w340) -> ("Flow Module Config"=w339:T3)
        n120 = Unbundle By Name(w339) -> ("Load Count"=w342:i32)
        n121 = Increment(x=w342) -> (x+1=w343:i32)
        n122 = Bundle By Name(cluster=w339, "Load Count"=w343) -> (w337:T3)
        n123 = call "Flow Settings Dialog.vi"("error in (no error)"=w335, "Flow Module Config In"=w337) -> ("error out"=w336:errorcluster, "UI Refresh Needed?"=w334:bool, "Flow Module Config Out"=w333:T3)  [unwired: 6 in, 1 out]
        n124 = case shown="False" w334 {
          tunnel: w336 -> [w346 w349]
          tunnel: [w345 w349] -> w328
          tunnel: w341 -> [_ _]
          tunnel: w338 -> [w348 _]
          tunnel: w333 -> [_ _]
          frame False {
            n125 = call-poly "Enqueue Message.vi"("error in (no error)"=w346, "Message"="Broadcast Settings", "Message Queue"=w348) -> ("error out"=w345:errorcluster)  [unwired: 7 in, 1 out]
          }
          frame True {
          }
        }
        n126 = Bundle By Name(cluster=w340, "Flow Module Config"=w333) -> (w329:T2)
        n127 = Unbundle By Name(w329) -> ("Flow Module Config.Process Name"=w332:string)
        n128 = Concatenate Strings(w332, " Settings Dialog Launched" ("text")) -> (w330:string)
        n129 = call "Write to Log File.vi"("error in"=w328, "text"=w330) -> ()  [unwired: 9 in, 1 out]
      }
      frame "Logging Stopped" {
        # "Logic for determining what action to take when the logging has stopped."
        n130 = case shown="\"Waiting for Exit (Acq Stopped)\"" w358 {
          selector: w358 -> [w360 _ _ _ _]
          tunnel: [w360 UI_State."Waiting for Exit (Log Stopped)" ("UI State") UI_State."Waiting for Stop (Log Stopped)" ("UI State") UI_State."Idle" ("UI State") UI_State."Idle" ("UI State")] -> w357
          tunnel: w356 -> [w359 w361 w363 w369 w375]
          tunnel: [w359 w361 w363 w368 w374] -> w351
          tunnel: w355 -> [_ _ _ w367 w373]
          frame Default {
          }
          frame "Waiting for Exit", "Waiting for Exit (Log Stopped)" {
          }
          frame "Waiting for Stop", "Waiting for Stop (Log Stopped)" {
          }
          frame "Waiting for Exit (Acq Stopped)" {
            # "If we are waiting to exit, and the acquisition has already stopped, then the \"Logging Stopped\" message indicates that it is time to exit."
            n131 = call-poly "Enqueue Message.vi"("Priority Message? (F)"=TRUE, "error in (no error)"=w369, "Message"="Exit", "Message Queue"=w367) -> ("error out"=w368:errorcluster)  [unwired: 6 in, 1 out]
          }
          frame "Waiting for Stop (Acq Stopped)" {
            # "If we are waiting to stop, and the acquisition has already stopped, then the \"Logging Stopped\" message indicates that it is time to stop."
            n132 = call-poly "Enqueue Message.vi"("error in (no error)"=w375, "Message Data"="Ready..." ("Message"), "Message"="Update Status", "Message Queue"=w373) -> ("error out"=w374:errorcluster)  [unwired: 6 in, 1 out]
          }
        }
        n133 = Unbundle By Name(w350) -> ("Flow Module Config.Process Name"=w354:string)
        n134 = Concatenate Strings(w354, " Logging Stopped" ("text")) -> (w352:string)
        n135 = call "Write to Log File.vi"("error in"=w351, "text"=w352) -> ()  [unwired: 9 in, 1 out]
      }
      frame "Start" {
        # "There is only one loop but i am keeping it in for now"
        # "Message Acquisition and Logging loops to start"
        # "Start - Enable/Disable buttons appropriately for an acquisition that has started, and update status display."
        n136 = call-poly "Enqueue Message.vi"("error in (no error)"=w382, "Message"="Start Loops", "Message Queue"=w383) -> ("error out"=w384:errorcluster)  [unwired: 7 in, 1 out]
        n137 = Merge Errors(w384) -> (w378:errorcluster)
        n138 = Unbundle By Name(w377) -> ("Flow Module Config.Process Name"=w381:string)
        n139 = Concatenate Strings(w381, " Start" ("text")) -> (w379:string)
        n140 = call "Write to Log File.vi"("error in"=w378, "text"=w379) -> ()  [unwired: 9 in, 1 out]
      }
      frame "Start Loops" {
        # "I'm not sure how you could have multiple Process names in one Module"
        # "Message Acquisition and Logging loops to start"
        # "Start - Enable/Disable buttons appropriately for an acquisition that has started, and update status display."
        n141 = Unbundle By Name(w387) -> ("Flow Module Config.Process Name"=w388:string)
        n142 = Build Array(w392) -> (w390:refnum<queue>[])
        n143 = property class="VI"("Front Panel.Title"=w388) -> ()  [unwired: 2 in, 2 out]
        n144 = for {
          tunnel: w389 -> [w398]
          tunnel: [w397] -> w391 mode=indexing
          tunnel: w390 -> [w396] mode=indexing
          tunnel: w388 -> [w395]
          n145 = call-poly "Enqueue Message.vi"("error in (no error)"=w398, "Message Data"=w395, "Message"="Start", "Message Queue"=w396) -> ("error out"=w397:errorcluster)  [unwired: 6 in, 1 out]
        }
        n146 = Merge Errors(w391) -> (w394:errorcluster)
      }
      frame "Start Log" {
        # "Message Acquisition and Logging loops to start"
        # "Start - Enable/Disable buttons appropriately for an acquisition that has started, and update status display."
        n147 = call-poly "Enqueue Message.vi"("error in (no error)"=w408, "Message Data"=w405, "Message"="Start Log", "Message Queue"=w406) -> ("error out"=w409:errorcluster)  [unwired: 6 in, 1 out]
        n148 = Merge Errors(w409) -> (w401:errorcluster)
        n149 = Unbundle By Name(w400) -> ("Flow Module Config.Process Name"=w404:string)
        n150 = Concatenate Strings(w404, " Start Log" ("text")) -> (w402:string)
        n151 = call "Write to Log File.vi"("error in"=w401, "text"=w402) -> ()  [unwired: 9 in, 1 out]
      }
      frame "Stop" {
        # "Stop - Enable/Disable buttons appropriately for an acquisition that has stopped, and update status display."
        n152 = call-poly "Enqueue Message.vi"("error in (no error)"=w420, "Message Data"="Ready..." ("Ready..."), "Message"="Update Status", "Message Queue"=w425) -> ("error out"=w418:errorcluster)  [unwired: 6 in, 1 out]
        n153 = call-poly "Enqueue Message.vi"("error in (no error)"=w418, "Message"="Stop", "Message Queue"=w419) -> ("error out"=w416:errorcluster)  [unwired: 7 in, 1 out]
        n154 = case shown="Default" w421 {
          selector: w421 -> [_ w427]
          tunnel: [UI_State."Waiting for Stop" ("UI State") w427] -> w422
          frame Default {
          }
          frame "Waiting for Exit" {
          }
        }
        n155 = Merge Errors(w416) -> (w412:errorcluster)
        n156 = Unbundle By Name(w411) -> ("Flow Module Config.Process Name"=w415:string)
        n157 = Concatenate Strings(w415, " Stop" ("text")) -> (w413:string)
        n158 = call "Write to Log File.vi"("error in"=w412, "text"=w413) -> ()  [unwired: 9 in, 1 out]
      }
      frame "Update Status" {
        # "Update Display - Convert the message data to a string to display in the Status indicator."
        n159 = Variant To Data(error in=w434, type="", Variant=w433) -> (data=→"Status":string, error out=w431:errorcluster)
        n160 = Merge Errors(w431) -> (w435:errorcluster)
      }
      frame Default {
        # "'Default' case only runs if there is a message that isn't defined in any of the other cases.  Output a programming error."
        n161 = Concatenate Strings("The invalid message string " ("string"), w436, " was received in Feed Module Main." ("string")) -> (w438:string)
        n162 = Bundle By Name(cluster=errorcluster {"status"=TRUE, "code"=1, "source"=""} ("error constant"), "source"=w438) -> (w437:errorcluster)
        n163 = Unbundle By Name(w442) -> ("Flow Module Config.Process Name"=w445:string)
        n164 = Concatenate Strings(w445, "Incorrect Message recieved: " ("text"), w436) -> (w443:string)
        n165 = call "Write to Log File.vi"("error in"=w437, "text"=w443) -> ()  [unwired: 9 in, 1 out]
      }
    }
    n166 = call "Error Handler - Message Handling Loop.vi"("error in (no error)"=w103, "Message Queue"=w101) -> ("dup error in"=w102:errorcluster)  [unwired: 8 in, 1 out]
  }
  n167 = call "Main Loop.vi"("error in (no error)"=w7, "Chart Notifier"=w20, "Message Queues"=w6) -> ("error out"=w21:errorcluster)  [unwired: 8 in]
  n168 = Close Reference(reference=w19) -> ()  [unwired: 1 in, 1 out]
  n169 = Unregister For Events(event registration refnum=w28, error in=w33) -> (error out=w29:errorcluster)
  n170 = Merge Errors(w29, w34, w7, w21) -> (w32:errorcluster)
  n171 = call "Destroy User Event - Stop.vi"("error in (no error)"=w32, "User Event - Stop"=w30) -> ("error out"=w3:errorcluster)  [unwired: 9 in]
  n172 = flat-sequence {
    tunnel: w3 -> [_]
    frame #0 {
      n173 = invoke class="VI" method="FP.Close"() -> ()  [unwired: 3 in, 3 out]
    }
  }
